vi "Read Capabilities.vi"(8 "error in (no error)":errorcluster, 11 "SLSC Switch in":refnum<class "SLSC Switch.lvclass">) -> (0 "error out":errorcluster, 2 "capabilities":string)   [LabVIEW 2015, in "SLSC Switch.lvlib" / "SLSC Switch.lvclass"]
uses:
  SLSC Switch.lvclass
  SLSC Switch.lvclass/SLSC Switch.ctl
  <vilib>/SLSC/Initialize Session with NVMEM Areas.vi
  <vilib>/SLSC/Close Session.vi
  <vilib>/SLSC/SLSC.lvlib
  <resource>/objmgr/slsc.rc
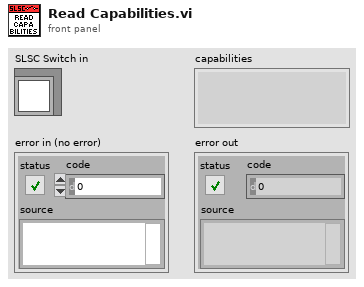
[diagram p1: front panel]
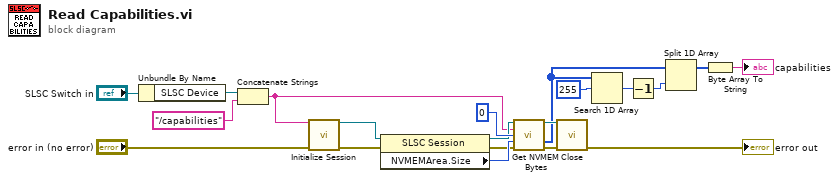
[diagram p0: block diagram]
diagram:
  n1 = Unbundle By Name("SLSC Switch in") -> ("SLSC Device"=w2:refnum<k21>)
  n2 = Concatenate Strings(w2, "/capabilities" ("string")) -> (w10:string)
  n3 = call-poly <vilib>:"Initialize Session.vi"("NVMEM areas"=w10, "error in (no error)"="error in (no error)") -> ("session out"=w11:refnum<k21>, "error out"=w12:errorcluster)  [unwired: 12 in]
  n4 = property class="SLSC Session"(reference=w11, error in=w12) -> (reference out=w15:refnum<k21>, error out=w14:errorcluster, "NVMEMArea.Size"=w17:u32)
  n5 = call <vilib>:"Get NVMEM Bytes.vi"("session in"=w15, "NVMEM area"=w10, "data address"=u32 0, "data size"=w17, "error in (no error)"=w14) -> ("session out"=w9:refnum<k21>, "data out"=w6:u8[], "error out"=w8:errorcluster)  [unwired: 6 in, 2 out]
  n6 = call-poly <vilib>:"Close.vi"("session in"=w9, "error in (no error)"=w8) -> ("error out"=→"error out":errorcluster)  [unwired: 13 in]
  n7 = Search 1D Array(1D array=w6, element=u8 255) -> (index of element=w4:i32)  [unwired: 1 in]
  n8 = Decrement(x=w4) -> (x-1=w3:i32)
  n9 = Split 1D Array(array=w6, index=w3) -> (first subarray=w5:u8[])  [unwired: 1 out]
  n10 = Byte Array To String(unsigned byte array=w5) -> (string=→"capabilities":string)
